vi "Path_Check.vi"(8 "Error In":errorcluster, 10 "Path In":path=path "C:/Users/X/Desktop/Materijali fakultet/LabVIEW/Diplomska/Virtuelen kalibrator/Programa/Main Programs/Logjgfjfgjfgjg.csv", 11 "Queue In":refnum<queue>) -> (0 "Error Out":errorcluster, 2 "Path Out":path=path "C:/Users/X/Desktop/Materijali fakultet/LabVIEW/Diplomska/Virtuelen kalibrator/Programa/Main Programs/Logjgfjfgjfgjg.csv", 3 "Queue Out":refnum<queue>)   [LabVIEW 2021, in "Main.lvlib" / "Main_Programs_SubVIs.lvlib"]
doc: "This VI is used to check the picked file type."
uses:
  Main_Programs_SubVIs.lvlib
  Tipski Definicii/Save_Sostojbi.ctl
  Polymorphic/Enq_Save_QMH.vi
  Polymorphic/Queues.lvlib
panel:
  # "Input"
  # "Output"
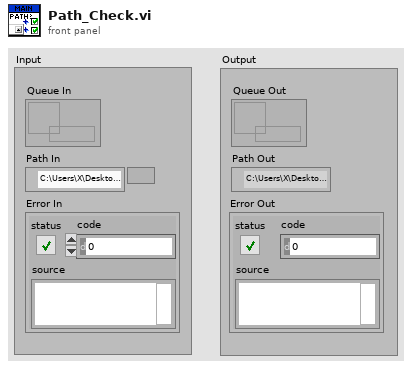
[diagram p1: front panel]
types:
  T1 = typedef "Save_Sostojbi.ctl" = enum16{"Init", "Generate Message", "Pick Path", "Save", "End"}
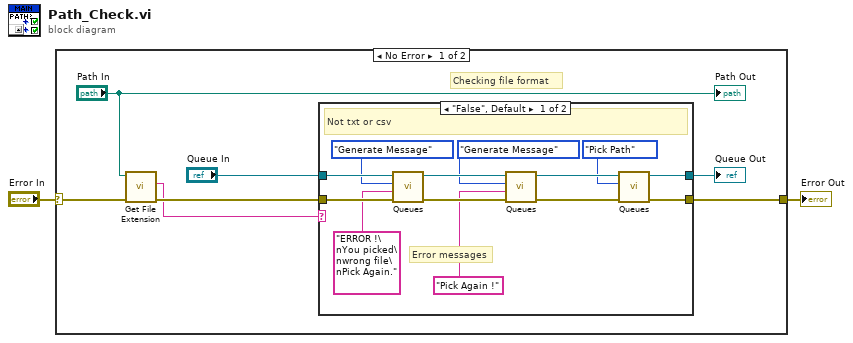
[diagram p0: block diagram]
diagram:
  n1 = case shown="No Error" "Error In" {
    selector: "Error In" -> [w6 w25]
    tunnel: [w8 w25] -> w1
    frame No Error {
      # "Checking file format"
      n2 = call <vilib>:"Get File Extension.vi"("error in (no error)"=w6, "file"="Path In") -> ("error out"=w5:errorcluster, "lowercase file extension"=w3:string)  [unwired: 5 in, 3 out]
      n3 = case shown="\"False\", Default" w3 {
        tunnel: w5 -> [w22 w24]
        tunnel: "Queue In" -> [w21 w23]
        tunnel: [w11 w24] -> w8
        tunnel: [w10 w23] -> w7
        frame "False", Default {
          # "Error messages"
          # "Not txt or csv"
          n4 = call-poly "Queues.vi"("Error In"=w22, "Message"="ERROR !\nYou picked\nwrong file\nPick Again.", "Instruction"=Save_Sostojbi."Generate Message", "Queue In"=w21) -> ("Error Out"=w18:errorcluster, "Queue Out"=w17:refnum<queue>)  [unwired: 6 in]
          n5 = call-poly "Queues.vi"("Error In"=w18, "Message"="Pick Again !", "Instruction"=Save_Sostojbi."Generate Message", "Queue In"=w17) -> ("Error Out"=w14:errorcluster, "Queue Out"=w13:refnum<queue>)  [unwired: 6 in]
          n6 = call-poly "Queues.vi"("Error In"=w14, "Instruction"=Save_Sostojbi."Pick Path", "Queue In"=w13) -> ("Error Out"=w11:errorcluster, "Queue Out"=w10:refnum<queue>)  [unwired: 7 in]
        }
        frame "csv", "ini", "txt" {
          # "csv,txt,ini"
        }
      }
      "Queue Out" <- w7
      "Path Out" <- "Path In"
    }
    frame Error {
    }
  }
  "Error Out" <- w1
